vi "Send Core OOB TX.vi"(8 "error in (no error)":errorcluster, 11 "CIFCorePlugin in":refnum<class "CIFCorePlugin.lvclass">) -> (0 "error out":errorcluster, 3 "CIFCorePlugin out":refnum<class "CIFCorePlugin.lvclass">)   [LabVIEW 2021, in "CIFCorePlugin.lvclass"]
uses:
  CIFCorePlugin.lvclass
  CIFCorePlugin.lvclass/CIFCorePlugin.ctl
  Channels/CIFChannelMng/CIFChannelMng.lvclass/CIFChannelMng.ctl
  Common/Typedef/Plugin Overrides.ctl
  Common/Typedef/Timing Overrides.ctl
  Common/Typedef/Plugin Status.ctl
  Common/Typedef/Plugin State.ctl
  Common/Typedef/Timing Statistics.ctl
  Common/Typedef/Timing Stats Base.ctl
  Common/Typedef/FIFO Statistics.ctl
  Common/Typedef/Simple Error.ctl
  Common/Typedef/Monitor Doubles.ctl
  Common/Typedef/Monitor U64.ctl
  Common/Typedef/Monitor I64.ctl
  CIFUtilities/CIFOutOfBand/CIFOutOfBand.lvclass/CIFOutOfBand.ctl
  CIFUtilities/CIFOutOfBand/Write OOB DVR.vi
  CIFUtilities/CIFOutOfBand/Utilities/Command to Bitwise Command.vi
  CIFUtilities/CIFOutOfBand/Accessors/Read Local OOB Data.vi
  CIFUtilities/CIFOutOfBand/Accessors/Write Local OOB Data.vi
  Channels/CIFChannelMng/Accessors/Read Update OOB.vi
  Channels/CIFChannelMng/Accessors/Read Channel Status for OOB.vi
  Channels/CIFChannelMng/Accessors/Write Update OOB.vi
  OOB/OOB_Tx/CIFCoreOOB_Tx.lvclass
  D:/dev/CIF-LVCore/src/CIFUtilities/CIFOutOfBand/CIFOutOfBand.lvclass
  Common/CIFCoreCommon.lvlib
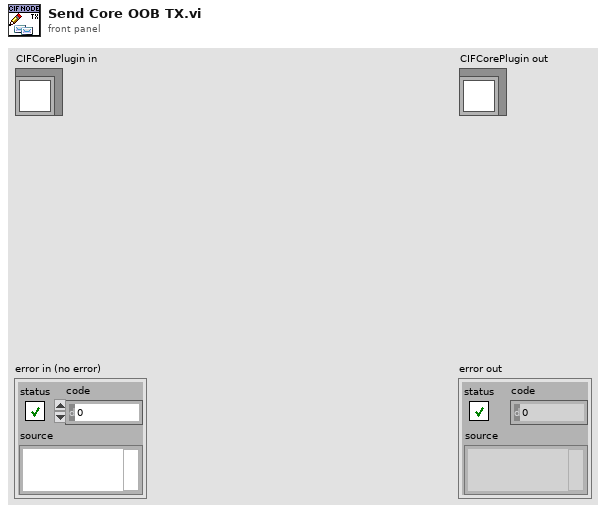
[diagram p1: front panel]
types:
  T1 = typedef "CIFCoreCommon.lvlib/Plugin Overrides.ctl" = cluster{"Timing Overrides":T2}
  T2 = typedef "CIFCoreCommon.lvlib/Timing Overrides.ctl" = cluster{"Override Timing":bool, "Skip Sleep":bool, "Period (s)":dbl}
  T3 = typedef "CIFCoreCommon.lvlib/Plugin Status.ctl" = cluster{"State":T4, "Timing Statistics (us)":T5, "FIFO Statistics (us)":T7, "error":T8, "Monitor Doubles":T9, "Monitor U64":T10, "Monitor I64":T11, "Cleanup":T6, "Create":i32, "Destroy":i32}
  T4 = typedef "CIFCoreCommon.lvlib/Plugin State.ctl" = enum32{"Null", "Creating", "Listening", "Running", "CleaningUp", "Destroying"}
  T5 = typedef "CIFCoreCommon.lvlib/Timing Statistics.ctl" = cluster{"Period":T6, "Wake Error":T6, "Execute":T6, "Housekeep":T6, "Idle":T6}
  T6 = typedef "CIFCoreCommon.lvlib/Timing Stats Base.ctl" = cluster{"Max":i32, "Min":i32}
  T7 = typedef "CIFCoreCommon.lvlib/FIFO Statistics.ctl" = cluster{"From T0":T6, "From Previous Plugin":T6, "Output Error":T6}
  T8 = typedef "CIFCoreCommon.lvlib/Simple Error.ctl" = cluster{"status":bool, "code":i32}
  T9 = typedef "CIFCoreCommon.lvlib/Monitor Doubles.ctl" = cluster{"1":dbl, "2":dbl, "3":dbl, "4":dbl}
  T10 = typedef "CIFCoreCommon.lvlib/Monitor U64.ctl" = cluster{"1":u64, "2":u64, "3":u64, "4":u64}
  T11 = typedef "CIFCoreCommon.lvlib/Monitor I64.ctl" = cluster{"1":i64, "2":i64, "3":i64, "4":i64}
  T12 = typedef "CIFChannelMng.lvclass/Channel List for OOB.ctl" = cluster{"Name":string, "Direction":T13, "Type":string, "Connected?":bool, "Connected Name":string, "Custom Config Data":u8[], "Forced?":bool}
  T13 = typedef "CIFChannels.lvclass/Direction.ctl" = enum16{"Publisher", "Subscriber"}
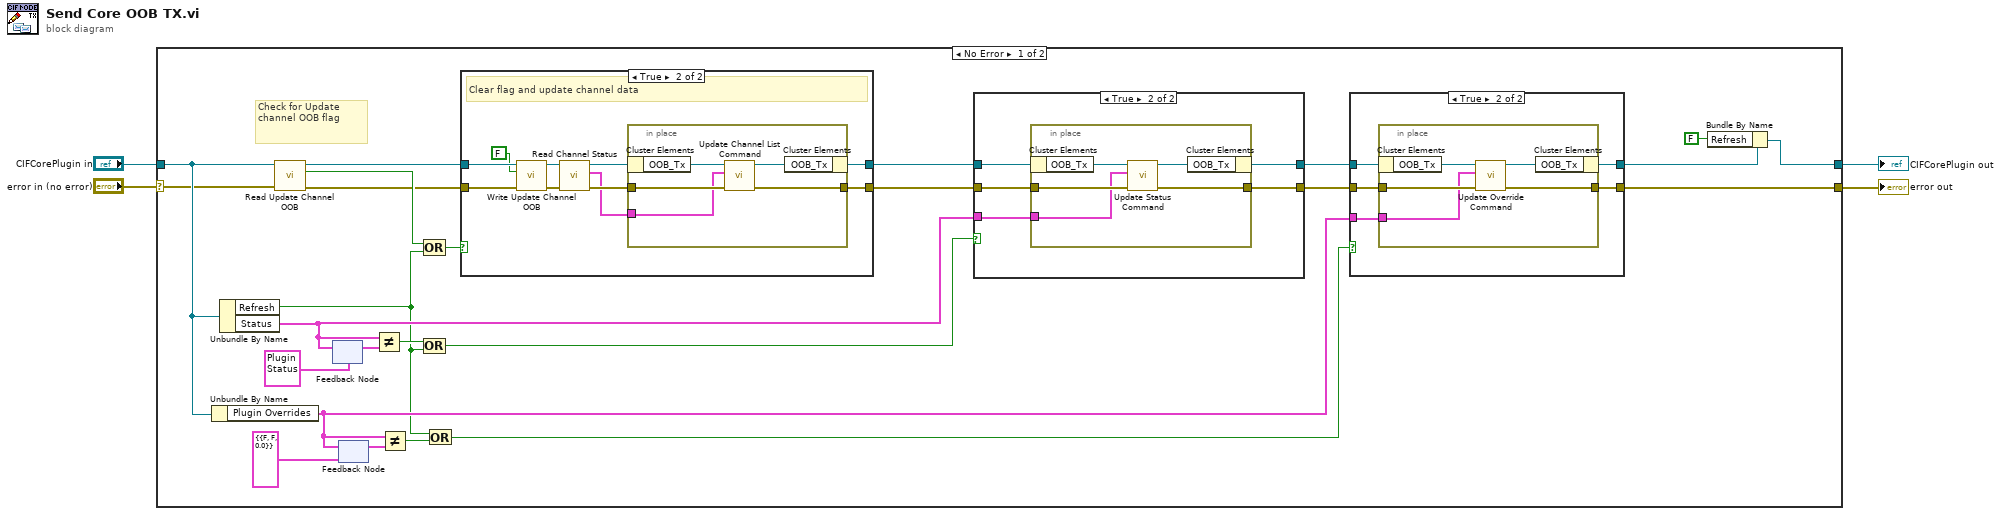
[diagram p0: block diagram]
diagram:
  n1 = case shown="No Error" "error in (no error)" {
    selector: "error in (no error)" -> [w12 w72]
    tunnel: [w9 w72] -> w3
    tunnel: [w5 w71] -> w1
    tunnel: "CIFCorePlugin in" -> [w15 w71]
    frame No Error {
      # "Check for Update channel OOB flag"
      n2 = Unbundle By Name(w15) -> ("Plugin Overrides"=w18:T1)
      n3 = Unbundle By Name(w15) -> ("Refresh"=w8:bool, "Status"=w26:T3)
      n4 = call "Read Update Channel OOB.vi"("error in (no error)"=w12, "CIFCorePlugin in"=w15) -> ("error out"=w11:errorcluster, "Update OOB"=w17:bool, "CIFCorePlugin out"=w13:refnum<class "CIFCorePlugin.lvclass">)  [unwired: 7 in]
      n5 = feedback-in #1(w26) -> ()
      n6 = feedback #1(T3 {"State"=enum."Null", "Timing Statistics (us)"={"Period"={"Max"=0, "Min"=0}, "Wake Error"={"Max"=0, "Min"=0}, "Execute"={"Max"=0, "Min"=0}, "Housekeep"={"Max"=0, "Min"=0}, "Idle"={"Max"=0, "Min"=0}}, "FIFO Statistics (us)"={"From T0"={"Max"=0, "Min"=0}, "From Previous Plugin"={"Max"=0, "Min"=0}, "Output Error"={"Max"=0, "Min"=0}}, "error"={"status"=FALSE, "code"=0}, "Monitor Doubles"={"1"=0.0, "2"=0.0, "3"=0.0, "4"=0.0}, "Monitor U64"={"1"=0, "2"=0, "3"=0, "4"=0}, "Monitor I64"={"1"=0, "2"=0, "3"=0, "4"=0}, "Cleanup"={"Max"=0, "Min"=0}, "Create"=0, "Destroy"=0} ("Status")) -> (w28:T3)
      n7 = feedback #2(T1 {"Timing Overrides"={"Override Timing"=FALSE, "Skip Sleep"=FALSE, "Period (s)"=0.0}} ("Plugin Overrides")) -> (w21:T1)
      n8 = feedback-in #2(w18) -> ()
      n9 = Not Equal?(x=w26, y=w28) -> (x != y?=w27:bool)
      n10 = Not Equal?(x=w18, y=w21) -> (x != y?=w22:bool)
      n11 = Compound Arithmetic op=OR(w17, w8) -> (w10:bool)
      n12 = Compound Arithmetic op=OR(w27, w8) -> (w25:bool)
      n13 = Compound Arithmetic op=OR(w8, w22) -> (w19:bool)
      n14 = case shown="True" w10 {
        tunnel: w11 -> [w30 w35]
        tunnel: w13 -> [w31 w36]
        tunnel: [w31 w41] -> w16
        tunnel: [w30 w40] -> w14
        frame False {
        }
        frame True {
          # "Clear flag and update channel data"
          n15 = call "Write Update Channel OOB.vi"("error in (no error)"=w35, "Update OOB"=FALSE, "CIFCorePlugin in"=w36) -> ("error out"=w33:errorcluster, "CIFCorePlugin out"=w34:refnum<class "CIFCorePlugin.lvclass">)  [unwired: 7 in]
          n16 = call "Read Channel Status.vi"("error in (no error)"=w33, "CIFCorePlugin in"=w34) -> ("error out"=w38:errorcluster, "Channel Status"=w37:T12[], "CIFCorePlugin out"=w39:refnum<class "CIFCorePlugin.lvclass">)  [unwired: 7 in]
          n17 = in-place {
            in-place-border: w38 -> [w44]
            in-place-border: [w43] -> w40
            in-place-border: w37 -> [w42]
            n18 = in-place-cluster #3(w39) -> ("OOB_Tx"=w46:refnum<class "CIFCoreOOB_Tx.lvclass">)
            n19 = call "Update Channel List Command.vi"("error in"=w44, "Channel List"=w42, "CoreOOB_Tx in"=w46) -> ("error out"=w43:errorcluster, "CoreOOB_Tx out"=w45:refnum<class "CIFCoreOOB_Tx.lvclass">)  [unwired: 7 in]
            n20 = in-place-cluster #3("OOB_Tx"=w45) -> (w41:refnum<class "CIFCorePlugin.lvclass">)
          }
        }
      }
      n21 = case shown="True" w25 {
        tunnel: w14 -> [w59 w65]
        tunnel: w16 -> [w60 w64]
        tunnel: w26 -> [_ w63]
        tunnel: [w60 w62] -> w24
        tunnel: [w59 w61] -> w23
        frame False {
        }
        frame True {
          n22 = in-place {
            in-place-border: w65 -> [w68]
            in-place-border: [w67] -> w61
            in-place-border: w63 -> [w66]
            n23 = in-place-cluster #4(w64) -> ("OOB_Tx"=w70:refnum<class "CIFCoreOOB_Tx.lvclass">)
            n24 = call "Update Status Command.vi"("error in"=w68, "Status"=w66, "CoreOOB_Tx in"=w70) -> ("error out"=w67:errorcluster, "CoreOOB_Tx out"=w69:refnum<class "CIFCoreOOB_Tx.lvclass">)  [unwired: 7 in]
            n25 = in-place-cluster #4("OOB_Tx"=w69) -> (w62:refnum<class "CIFCorePlugin.lvclass">)
          }
        }
      }
      n26 = case shown="True" w19 {
        tunnel: w23 -> [w47 w53]
        tunnel: w24 -> [w48 w52]
        tunnel: w18 -> [_ w51]
        tunnel: [w48 w50] -> w7
        tunnel: [w47 w49] -> w9
        frame False {
        }
        frame True {
          n27 = in-place {
            in-place-border: w53 -> [w56]
            in-place-border: [w55] -> w49
            in-place-border: w51 -> [w54]
            n28 = in-place-cluster #5(w52) -> ("OOB_Tx"=w58:refnum<class "CIFCoreOOB_Tx.lvclass">)
            n29 = call "Update Override Command.vi"("error in"=w56, "Plugin Overrides"=w54, "CoreOOB_Tx in"=w58) -> ("error out"=w55:errorcluster, "CoreOOB_Tx out"=w57:refnum<class "CIFCoreOOB_Tx.lvclass">)  [unwired: 7 in]
            n30 = in-place-cluster #5("OOB_Tx"=w57) -> (w50:refnum<class "CIFCorePlugin.lvclass">)
          }
        }
      }
      n31 = Bundle By Name(cluster=w7, "Refresh"=FALSE ("Running Internal Data.Refresh")) -> (w5:refnum<class "CIFCorePlugin.lvclass">)
    }
    frame Error {
    }
  }
  "error out" <- w3
  "CIFCorePlugin out" <- w1
